vi "AlliGator Highlight Image ROI in Phasor Plot.vi"(0 "Source Image in":T1, 1 "Image Sum":T1, 2 "Source Image ROI Mask":T1, 5 "Phasor Plot Image in":T1, 7 "ROI":T2, 9 "[Corrected] Complex Phasor Array":csg[][](array[numeric]), 11 "Error In":errorcluster, 12 "Overlay Color":u32(colorbox), 13 "Phasor Plot Display Range":cluster{"Min Value":dbl, "Max Value":dbl}={"Min Value"=0.0, "Max Value"=nan}) -> (4 "Source Image out":T1, 6 "Phasor Plot Image out":T1, 10 "CPU (s)":dbl, 15 "Error Out":errorcluster)   [LabVIEW 2021, in "AlliGator Phasor Plot.lvlib"]
doc: "Highlights the phasors in the Phasor Plot image that corrspond to pixels in the Source Image ROI."
uses:
  AlliGator Phasor Plot.lvlib
  <vilib>/vision/Image Controls.llb/IMAQ Image.ctl
  Palette/Image Palette Information.ctl
  Image/Image Display Palette Type.ctl
  Globals, Variables, Constants/AlliGator Variables List.ctl
  Settings/AlliGator Settings List.ctl
  Phasor Ratio/AlliGator Phasor Plot Reference Points.ctl
  40af3798-00bb-4b94-b92d-50ae21bc0bc0.vi
  Image/Global Rectangle Origin & Size.vi
  Variant/Variant to Data/Variant to Boolean.vi
  Variant/Variant to Data/Variant to I32.vi
  Image/Image Get Pixel Color.vi
  Image/Adjust Pixel Overlay Brightness.vi
  Globals, Variables, Constants/AlliGator Globals, Variables & Constants.lvlib
  Phasor Ratio/AlliGator Phasor Ratio.lvlib
  Image/Image.lvlib
  Source Image/AlliGator Source Image.lvlib
  <vilib>/vision/NI_Vision_Development_Module.lvlib
  Error/Error.lvlib
  Time/Time.lvlib
  ROIs/AlliGator ROIs.lvlib
  Settings/AlliGator Settings.lvlib
  Variant/Variant to Data/Variant to Data.lvlib
  Palette/Palette.lvlib
panel:
  # "see the AlliGator License on the block diagram (Ctrl+E or Window:Show Block Diagram)"
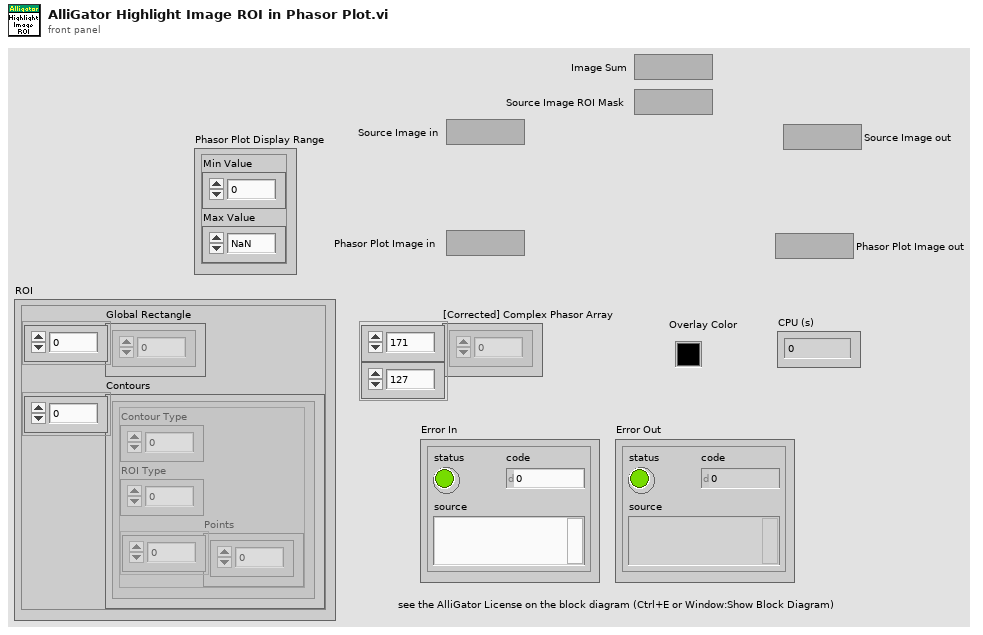
[diagram p1: front panel]
types:
  T1 = typedef "IMAQ Image.ctl" = refnum<image>
  T2 = cluster{"Global Rectangle":i32[], "Contours":cluster{"Contour Type":u32, "ROI Type":u32, "Points":i32[]}[]}
  T3 = typedef "Palette.lvlib/Image Palette Information.ctl" = cluster{"Palette Name [# Colors,int?,inv?]":string, "Palette Type":T4, "Palette Colors":u32[], "Interpolate?":bool}
  T4 = typedef "Image.lvlib/Image Display Palette Type.ctl" = u32
  T5 = typedef "AlliGator Globals, Variables & Constants.lvlib/AlliGator Variables List.ctl" = enum16{"---- GUI ----", "GUI:Initialization Status", "GUI:State Indicators Refnum", "GUI:Original AlliGator Menu Items", "GUI:Current Action Loop State", "GUI:Script in progress", "GUI:Playback", "GUI:Loop Playback", "GUI:Search ROI Used", "GUI:Search ROI", "Decay Graph Max Legend Size", "Intensity Graph Max Legend Size", "Decay Statistics Graph Max Legend Size", "Phasor Graph Max Legend Size", "Phasor Ratio Graph Max Legend Size", "Lifetime Graph Max Legend Size", "---- Files ----", "Files:Export Dataset Frames as Individual Files", "Files:Show Batch Export Help Balloons", "Files:Frames in Dataset", "Files:ptu File Frame Start Indices", "Files:Current Frame in Dataset", "Files:Current Frame Timestamp", "Files:Dataset Loaded", "Files:Dataset Metadata", "Files:Dataset Channel", "Files:Dataset Data Description", "Files:Background Dataset Metadata", "Files:Background Dataset Channel", "Files:Background Dataset Data Description", "Files:Background File Subtraction", "Files:Background File Path", "Files:Background File Pile-up Correction", "Files:Background File Pixel Well Capacity", "Files:Background File Scaling Factor", "Files:Current Dataset Load Settings", "Files:Dataset Path", "Files:ICCD-specific Information", "Files:Macrotime Gate Separation", "------ Python Plugins ------", "Python Plugins:Information", "Python Plugins:Python Session", "Python Plugins:Valid Python Session?", "---- Source Image ----", "Source Image:ROIs", "Source Image:Current ROI", "Source Image:ROI Event Refnum", "X_Source Image Display Range", "X_Source Image Palette Information", "X_Type of Displayed Image", "X_Time Gate Slider", "Source Image:Palette List", "Source Image:Scale", "Source Image:ROI Overlay Color", "Source Image:Overlay to Erase", "Source Image:Is Displayed Image Accumulated", "Source Image:White Light Image Modified", "Source Image:Mask Image Modified", "---- Image Profile Window ----", "Image Profile:Window Event Refnum", "Image Profile:IntensityType", "Image Profile:Intensity Average Type", "Image Profile:Intensity-weighted SDV", "Image Profile:Box Profile Type", "Image Profile:Window Open", "Image Profile:Plotted Fit Parameter", "------ Phasor Graph -------", "Phasor Graph:Show Line", "---- Phasor Plot ---", "Phasor Plot:Parameters Changed", "Phasor Plot:FLI Dataset Modified since last Calculation", "Phasor Harmonics Data", "Selected Phasor Harmonics", "Phasor Harmonic Manager Event Refnum", "Phasor Plot:ROIs", "Phasor Plot:Current ROI", "Phasor Plot:ROI Event Refnum", "Phasor Plot:Image Reference Points", "Phasor Plot:Computed", "Phasor Plot:Palette Information", "Phasor Plot:Palette List", "Phasor Plot:Phasor Ratio Palette Information", "Phasor Plot:Phasor Ratio Palette List", "Phasor Plot:Image Scale", "Phasor Plot:Image Overlay to Erase", "Phasor Plot:Image Elements to Update", "Phasor Plot:Current Calculation Parameters", "Phasor Plot:Current Calibration Options", "Phasor Plot:Reset Cumulated Phasor Plot", "Phasor Plot:Reference 1", "Phasor Plot:Lifetime Reference 1", "Phasor Plot:Reference 1 Frequency", "Phasor Plot:Reference 2", "Phasor Plot:Lifetime Reference 2", "Phasor Plot:Reference 2 Frequency", "---- Decay Analysis ----", "Number of Selected Decays to Fit", "LS Fit Results", "LAR Fit Results", "BS Fit Results", "Last Decay Max - Min", "Best Fit Parameters", "Best Fit Parameter Names", "Actual Size X", "Actual Size Y", "Binning X", "Binning Y", "Actual # Gates", "Dataset Number", "Gates to...", "Gates Skipped", "Gates to keep", "Gate Step", "Gate Separation", "Reversed Gates", "Pile-up Correction", "Pixel Well Capacity", "Background Subtracted", "Background Subtraction Method", "Background Definition Range", "Background File (deprecated)", "Number of Dataset Accumulated", "Array of Accumulated Dataset Paths", "Do Averaged Datasets", "Destination File Path", "Process Plot Target", "Use 1/D as Phasor Frequency", "---- Decay Fit Parameter Map -----", "Decay Fit Parameter Map:Palette Information", "Decay Fit Parameter Map:Palette List", "---- Parameter Map ----", "Parameter Map:Palette Information", "Parameter Map:Palette List", "------- Local Decay Window ---------", "Local Decay Graph Window:Event Refnum", "Local Decay Graph Window:Use normalized IRF for convolution", "----- Miscellaneous ----", "Misc:Skippable Dialog Windows Status"}
  T6 = typedef "AlliGator Settings.lvlib/AlliGator Settings List.ctl" = enum16{"GUI:Visible Settings Tab", "GUI:Last Run Version", "Source Image:Use Image Histogram for Contrast", "Source Image:Low Count Pixels Rejection Options", "Source Image:High Count Pixels Rejection Options", "Source Image:Use Image Brightness", "Source Image:Blend Overlay with Image Background", "Source Image:Use Fixed ROI Diameter", "Source Image:ROI Diameter", "Source Image:ROI Center Color", "Source Image:Peak Threshold", "Source Image:Intensity Threshold", "Source Image:Image Binning Options", "Source Image:Image Smoothing Options", "Source Image:Image Histogram Active", "Source Image:Invert Binary Mask", "Source Image:Hot Pixel Removal", "Source Image:Overlay Analyzed ROI Center", "Source Image:Auto-Adjust Contrast", "Source Image:Histogram Lower Percentile", "Source Image:Histogram Upper Percentile", "Source Image:Save Source Image", "Source Image:Scale Bar Options", "Source Image:Image Resolution (Pixel Size)", "Source Image:Flatfield Correction", "Source Image:Show Dead Left Columns Correction", "Source Image:Dead Left Columns Correction", "Source Image:Image Pre-Processing Operations Order", "Source Image:Overlay ROI Median", "Source Image:Median Overlay Color", "Data Information:Gate Width", "Data Information:Nanotime Gate Separation", "Data Information:Macrotime Gate Separation", "Data Information:Gate Step", "Data Information:# Gates", "Data Information:Gate Image Exposure", "Data Information:Gate Image Integration", "Data Information:Gates to Skip", "Data Information:Gates to Keep", "Data Information:Define Gates to", "Data Information:Channel Name", "Data Information:Available Channel Names", "Data Information:Channel Arithmetic", "Data Information:Background File Subtraction", "Data Information:Background File", "Data Information:Background Scaling Factor", "Data Information:Background Pile-up Correction", "Data Information:Background Pixel Well Capacity", "Data Information:Laser Period", "Data Information:SYNC Period", "Data Information:Pile-up Correction", "Data Information:Pixel Well Capacity", "Data Information:Dataset Scaling Factor", "Fluorescence Decay_Decay Pre-Processing:Reverse Gates", "Fluorescence Decay_Decay Pre-Processing:Verbose Decay Pre-Processing", "Fluorescence Decay_Decay Pre-Processing:Use Decay Pre-Processing", "Fluorescence Decay_Decay Pre-Processing:Background Subtraction", "Fluorescence Decay_Decay Pre-Processing:Background Definition Range", "Fluorescence Decay_Decay Pre-Processing:Baseline Subtraction Method", "Fluorescence Decay_Decay Pre-Processing:Decay Pre-Processing Operations Order", "Fluorescence Decay_Decay Pre-Processing:Smoothing Parameter", "Fluorescence Decay_Decay Pre-Processing:Shift Decay", "Fluorescence Decay_Decay Pre-Processing:Decay Shift Parameters", "Fluorescence Decay_Decay Pre-Processing:Fold Decay", "Fluorescence Decay_Decay Pre-Processing:# Folds", "Fluorescence Decay_Decay Pre-Processing:1-Normalize Decay", "Fluorescence Decay_Decay Pre-Processing:[0-1]-Normalize Decay", "Fluorescence Decay_Decay Pre-Processing:Smoothen Decay", "Fluorescence Decay_Decay Pre-Processing:Extrapolate Decay", "Fluorescence Decay_Decay Pre-Processing:Use Periodicity", "Fluorescence Decay_Decay Pre-Processing:Use Cursors", "Fluorescence Decay_Decay Pre-Processing:Tail Fraction", "Fluorescence Decay_Decay Pre-Processing:Head Fraction", "Fluorescence Decay_Decay Pre-Processing:Additional Points", "Fluorescence Decay_Decay Pre-Processing:Straighten Decay", "Fluorescence Decay_Decay Pre-Processing:Constant Background", "Fluorescence Decay_Decay Pre-Processing:Pixel-Normalize Decay", "Fluorescence Decay_Advanced Analysis:Extract IRF instead of Decay", "Fluorescence Decay_Advanced Analysis:IRF Extraction Options", "Fluorescence Decay_Advanced Analysis:IRF Optimization Options", "Fluorescence Decay_Advanced Analysis:Square Pulse Options", "Fluorescence Decay_Advanced Analysis:IRF Order", "Fluorescence Decay_Advanced Analysis:IRF Time Constants", "Fluorescence Decay_Advanced Analysis:Wavelet Analysis Options", "Fluorescence Decay_Advanced Analysis:Average Lifetime Options", "Fluorescence Decay_Fit Options:Fit Options", "Fluorescence Decay_Fit Options:Use Legacy Fitting Approach", "Fluorescence Decay_Fit Options:Use Data Information Laser Period", "Fluorescence Decay_Fit Parameters:Displayed Fit Parameters", "Fluorescence Decay_Fit Parameters:Fit Parameter Constraints", "Fluorescence Decay_Fit Parameters:Export Tabulated Results", "Fluorescence Decay_Fit Parameters:MLE Baseline Offset Type", "Fluorescence Decay_Fit Parameters:MLE Baseline Offset", "Fluorescence Decay_Fit Parameters:Guess Parameter Names", "Fluorescence Decay_Fit Parameters:Guess Parameter Values", "Fluorescence Decay_Fit Parameters:Guess Parameters Options", "Fluorescence Decay_Styles:Show Last Decay Only", "Fluorescence Decay_Styles:Decay Graph Color Array", "Fluorescence Decay:Decay Graph Active", "Fluorescence Decay Statistics:Min Peak Value", "Fluorescence Decay Statistics:Reject Low Decay Peak Pixels", "Fluorescence Decay Statistics:Reject High Decay Peak Pixels", "Fluorescence Decay Statistics:Max Peak Value", "Time Traces:Use File Timestamp", "Time Traces:Time Step", "Time Traces:Use Intensity Correction File", "Time Traces:Intensity Correction File", "Phasor Plot:Phasor Plot Smoothing Options", "Phasor Plot:Phasor Plot Size", "Phasor Plot:Phasor Plot Graphics Options", "Phasor Plot:Cumulative Phasor Plot", "Phasor Plot:Use Phasor Brightness", "Phasor Plot:Blend Overlay with Phasor Background", "Phasor Plot:Save Phasor Plot", "Phasor Plot:Show References", "Phasor Plot:Phasor Ratio Decay Range", "Phasor Plot:Exponential Fading", "Phasor Plot:Phasor Ratio Reference Colors", "Phasor Plot:Reference Radius", "Phasor Plot:Show Color Map Vertices", "Phasor Plot:Phasor Plot Active", "Phasor Plot:Phasor Ratio Color Map Type", "Phasor Plot:Phasor Ratio Color Map", "Phasor Plot:Phasor Ratio Display Range", "Phasor Plot:Selected Image ROI(s)", "Phasor Plot:All Image ROIs", "Phasor Plot:Selected Phasor Plot ROI(s)", "Phasor Plot:All Phasor Plot ROIs", "Phasor Plot:Phasor Ratio Color-Coded Quantity", "Phasor Plot:Store Phasor Harmonics", "Phasor Plot:Draw Reference Segment", "Phasor Plot:User-Defined Quantity", "Phasor Graph:Phasor Frequency", "Phasor Graph:Phasor Ratio Type", "Phasor Graph:Pixel-level Phasor Computation", "Phasor Graph:Save Phasor Graph", "Phasor Graph:Phasor Graph Active", "Phasor Graph:Phasor SDV Options", "Phasor Calibration:Use Backup Calibration if needed", "Phasor Graph:Define Shortest Lifetime as", "Phasor Calibration:Backup Calibration Type", "Phasor Calibration:Calibration Type", "Phasor Calibration:Calibration Lifetime", "Phasor Calibration:Calibration Map Algorithm", "Single-Exponential Phasor Locus (SEPL):Gate Parameters", "Single-Exponential Phasor Locus (SEPL):User-defined Gate", "Single-Exponential Phasor Locus (SEPL):User-defined IRF", "Single-Exponential Phasor Locus (SEPL):Phasor Parameters", "Single-Exponential Phasor Locus (SEPL):Decay & IRF Parameters", "Single-Exponential Phasor Locus (SEPL):Display Parameters", "Lifetime Analysis:Decay Analysis Parameters", "Lifetime Analysis:Lifetime Map Active", "Plugins:Python Settings", "Miscellaneous:Verbose Mode", "Miscellaneous:Beep after Script", "Miscellaneous:Saved Image File Format", "Miscellaneous:Exported Gate Image Settings", "Miscellaneous:Include Loading in Timing", "Miscellaneous:Verbose Settings Mode", "Miscellaneous:Histogram Options", "Miscellaneous:Beep on Error", "Miscellaneous:# Logical Processors Used", "Miscellaneous:ROI Description Max Characters", "Miscellaneous:Verbose Error Mode", "Miscellaneous:Transparent Mask Color"}
  T7 = typedef "AlliGator Phasor Ratio.lvlib/AlliGator Phasor Plot Reference Points.ctl" = cluster{"O_h":dbl, "O_v":dbl, "1_h":dbl, "1_v":dbl}
  T8 = typedef "ROI Descriptor" = cluster{"Global Rectangle":i32[], "Contours":cluster{"ID":enum32{"External", "Internal"}, "Type":u32, "Coordinates":i32[]}[]}
  T9 = cluster{"Red (or Hue) value":u8, "Green (or Sat) value":u8, "Blue (or Light or Val) value":u8}
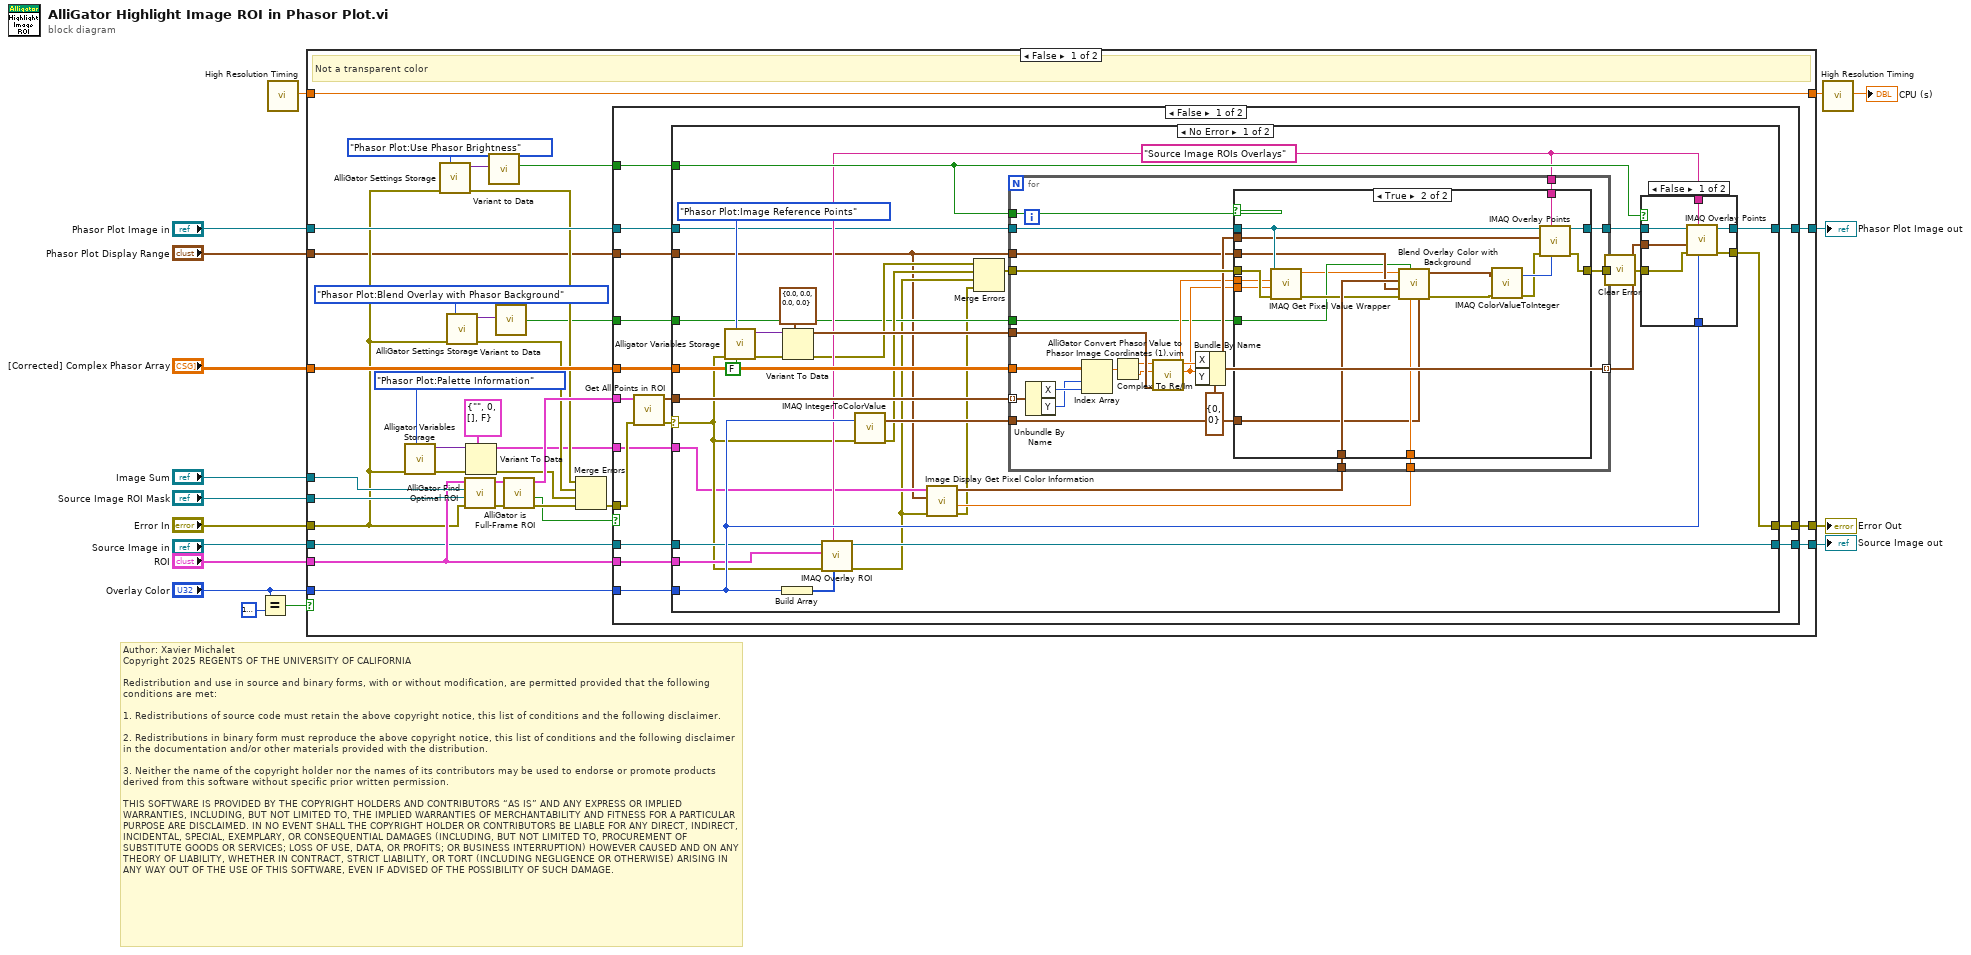
[diagram p0: block diagram]
diagram:
  # "Author: Xavier Michalet\nCopyright 2025 REGENTS OF THE UNIVERSITY OF CALIFORNIA\n\nRedistribution and use in source and binary forms, with or without modification, are permitted provided that the following conditions are met:\n\n1. Redistributions of source code must retain the above copyright notice, this list of conditions and the following disclaimer.\n\n2. Redistributions in binary form must reproduce the above copyright notice, this list of conditions and the following disclaimer in the documentation and/or other materials provided with the distribution.\n\n3. Neither the name of the copyright holder nor the names of its contributors may be used to endorse or promote products derived from this software without specific prior written permission.\n\nTHIS SOFTWARE IS PROVIDED BY THE COPYRIGHT HOLDERS AND CONTRIBUTORS “AS IS” AND ANY EXPRESS OR IMPLIED WARRANTIES, INCLUDING, BUT NOT LIMITED TO, THE IMPLIED WARRANTIES OF MERCHANTABILITY AND FITNESS FOR A PARTICULAR PURPOSE ARE DISCLAIMED. IN NO EVENT SHALL THE COPYRIGHT HOLDER OR CONTRIBUTORS BE LIABLE FOR ANY DIRECT, INDIRECT, INCIDENTAL, SPECIAL, EXEMPLARY, OR CONSEQUENTIAL DAMAGES (INCLUDING, BUT NOT LIMITED TO, PROCUREMENT OF SUBSTITUTE GOODS OR SERVICES; LOSS OF USE, DATA, OR PROFITS; OR BUSINESS INTERRUPTION) HOWEVER CAUSED AND ON ANY THEORY OF LIABILITY, WHETHER IN CONTRACT, STRICT LIABILITY, OR TORT (INCLUDING NEGLIGENCE OR OTHERWISE) ARISING IN ANY WAY OUT OF THE USE OF THIS SOFTWARE, EVEN IF ADVISED OF THE POSSIBILITY OF SUCH DAMAGE."
  n1 = Equal?(x="Overlay Color", y=u32 16777216 ("Overlay Color")) -> (x = y?=w10:bool)
  n2 = call "High Resolution Timing.vi"() -> ("elapsed (relative) seconds"=w12:dbl)  [unwired: 17 in, 2 out]
  n3 = case shown="False" w10 {
    tunnel: "[Corrected] Complex Phasor Array" -> [w50 _]
    tunnel: "Error In" -> [w22 w162]
    tunnel: [w38 w162] -> w15
    tunnel: "Image Sum" -> [w49 _]
    tunnel: "Overlay Color" -> [w48 _]
    tunnel: w12 -> [w47 w161]
    tunnel: [w47 w161] -> w11
    tunnel: "Source Image ROI Mask" -> [w46 _]
    tunnel: "Phasor Plot Image in" -> [w43 w160]
    tunnel: [w42 w160] -> w6
    tunnel: "ROI" -> [w41 _]
    tunnel: "Source Image in" -> [w40 w159]
    tunnel: [w39 w159] -> w3
    tunnel: "Phasor Plot Display Range" -> [w18 _]
    frame False {
      # "Not a transparent color"
      n4 = call "Alligator Variables Storage.vi"("AlliGator Variable"=AlliGator_Variables_List."Phasor Plot:Palette Information" ("Alligator Variable"), "Error In"=w22) -> ("Error Out"=w21:errorcluster, "Data out"=w25:variant)  [unwired: 7 in, 1 out]
      n5 = call "AlliGator Settings Storage.vi"("AlliGator Settings List"=AlliGator_Settings_List."Phasor Plot:Use Phasor Brightness", "Error In"=w22) -> ("Error Out"=w31:errorcluster, "Variant Data out"=w34:variant)  [unwired: 8 in]
      n6 = call "AlliGator Settings Storage.vi"("AlliGator Settings List"=AlliGator_Settings_List."Phasor Plot:Blend Overlay with Phasor Background", "Error In"=w22) -> ("Error Out"=w27:errorcluster, "Variant Data out"=w28:variant)  [unwired: 8 in]
      n7 = call "AlliGator Find Optimal ROI.vi"("error in (no error)"=w22, "ROI Mask"=w46, "Image Sum"=w49, "ROI Descriptor in"=w41) -> ("error out"=w45:errorcluster, "ROI Descriptor out"=w44:T8)  [unwired: 5 in, 1 out]
      n8 = Variant To Data(error in=w21, type=T3 {"Palette Name [# Colors,int?,inv?]"="", "Palette Type"=0, "Palette Colors"=[], "Interpolate?"=FALSE} ("Image Display Palette Information"), Variant=w25) -> (data=w19:T3, error out=w20:errorcluster)
      n9 = call-poly "Variant to Data.vi"("Variant"=w34) -> ("Value"=w33:bool)  [unwired: 8 in]
      n10 = call-poly "Variant to Data.vi"("Variant"=w28) -> ("Value"=w26:bool)  [unwired: 8 in]
      n11 = call "AlliGator is Full-Frame ROI.vi"("error in (no error)"=w45, "ROI Descriptor in"=w44) -> ("error out"=w37:errorcluster, "Full-Frame ROI?"=w35:bool, "ROI Descriptor (dup)"=w36:T8)  [unwired: 7 in]
      n12 = Merge Errors(w31, w27, w20, w37) -> (w32:errorcluster)
      n13 = case shown="False" w35 {
        tunnel: w50 -> [w66 _]
        tunnel: w33 -> [w65 _]
        tunnel: w48 -> [w64 _]
        tunnel: w43 -> [w61 w156]
        tunnel: [w60 w156] -> w42
        tunnel: w41 -> [w59 _]
        tunnel: w40 -> [w58 w157]
        tunnel: [w57 w157] -> w39
        tunnel: [w56 w158] -> w38
        tunnel: w32 -> [w55 w158]
        tunnel: w36 -> [w54 _]
        tunnel: w26 -> [w53 _]
        tunnel: w19 -> [w52 _]
        tunnel: w18 -> [w51 _]
        frame False {
          n14 = call "Get All Points in ROI.vi"("Error In"=w55, "ROI Descriptor"=w54) -> ("Error Out"=w62:errorcluster, "Point Array"=w63:cluster{"X":i32, "Y":i32}[])  [unwired: 8 in]
          n15 = case shown="No Error" w62 {
            selector: w62 -> [w74 _]
            tunnel: w66 -> [w100 _]
            tunnel: w65 -> [w99 _]
            tunnel: w64 -> [w98 _]
            tunnel: w59 -> [w97 _]
            tunnel: w63 -> [w89 _]
            tunnel: w61 -> [w79 w154]
            tunnel: [w78 w154] -> w60
            tunnel: w58 -> [w77 w155]
            tunnel: [w76 w155] -> w57
            tunnel: [w75 _] -> w56
            tunnel: w53 -> [w73 _]
            tunnel: w52 -> [w72 _]
            tunnel: w51 -> [w67 _]
            frame No Error {
              w84 = "Source Image ROIs Overlays" ("Group")
              n16 = call "Alligator Variables Storage.vi"("Get(F)/Set"=FALSE, "AlliGator Variable"=AlliGator_Variables_List."Phasor Plot:Image Reference Points" ("Alligator Variable"), "Error In"=w74) -> ("Error Out"=w92:errorcluster, "Data out"=w94:variant)  [unwired: 6 in, 1 out]
              n17 = Build Array(w98) -> (w90:u32[])
              n18 = Variant To Data(error in=w92, type=T7 {"O_h"=0.0, "O_v"=0.0, "1_h"=0.0, "1_v"=0.0} ("Phasor Plot Reference Points"), Variant=w94) -> (data=w91:T7, error out=w81:errorcluster)
              n19 = call "IMAQ Overlay ROI"("Colors (Green)"=w90, "Group"=w84, "error in (no error)"=w74, "ROI Descriptor"=w97, "Image"=w77) -> ("error out"=w69:errorcluster, "Image Out"=w76:T1)  [unwired: 5 in]
              n20 = call "IMAQ IntegerToColorValue"("error in (no error)"=w74, "U32 value"=w98) -> ("error out"=w80:errorcluster, "Color Value"=w85:T9)  [unwired: 3 in, 2 out]
              n21 = call "Image Display Get Pixel Color Information.vi"("Error In"=w69, "Image Display Range"=w67, "Image Display Palette Information"=w72) -> ("Error Out"=w68:errorcluster, "Image Scale Factor (256 colors)"=w70:sgl, "1D Color Array"=w71:cluster{"Red":u8, "Green":u8, "Blue":u8}[])  [unwired: 5 in, 1 out]
              n22 = Merge Errors(w81, w80, w69, w68) -> (w82:errorcluster)
              n23 = for {
                tunnel: w100 -> [w132]
                tunnel: w91 -> [w131]
                tunnel: w89 -> [w129] mode=indexing
                tunnel: [w120] -> w88 mode=indexing
                tunnel: w99 -> [w125]
                tunnel: w85 -> [w114]
                tunnel: w84 -> [w119]
                tunnel: w82 -> [w122]
                tunnel: [w121] -> w86
                tunnel: w79 -> [w124]
                tunnel: [w123] -> w87
                tunnel: w73 -> [w113]
                tunnel: w71 -> [w112]
                tunnel: w70 -> [w111]
                tunnel: w67 -> [w110]
                n24 = Unbundle By Name(w129) -> ("X"=w116:i32, "Y"=w115:i32)
                n25 = Index Array(array=w132, index (row)=w115, index (col)=w116) -> (element=w130:csg)
                n26 = Complex To Re/Im(x + iy=w130) -> (x=w128:sgl, y=w127:sgl)
                n27 = call "AlliGator Convert Phasor Value to Phasor Image Coordinates (1).vim"("Phasor Plot Reference Points"=w131, "Phasor s"=w127, "Phasor g"=w128) -> ("Phasor Plot y"=w117:dbl, "Phasor Plot x"=w118:dbl)  [unwired: 7 in]
                n28 = Bundle By Name(cluster=cluster{"X":i32, "Y":i32} {"X"=0, "Y"=0} ("Point"), "X"=w118, "Y"=w117) -> (w120:cluster{"X":i32, "Y":i32})
                n29 = case shown="True" w125 {
                  tunnel: w124 -> [w134 w151]
                  tunnel: [w134 w153] -> w123
                  tunnel: w122 -> [w133 w152]
                  tunnel: [w133 w147] -> w121
                  tunnel: w120 -> [_ w150]
                  tunnel: w119 -> [_ w146]
                  tunnel: w118 -> [_ w145]
                  tunnel: w117 -> [_ w144]
                  tunnel: w114 -> [_ w137]
                  tunnel: w113 -> [_ w139]
                  tunnel: w112 -> [_ w143]
                  tunnel: w111 -> [_ w138]
                  tunnel: w110 -> [_ w142]
                  frame False {
                  }
                  frame True {
                    n30 = call "IMAQ Get Pixel Value Wrapper.vi"("Error In"=w152, "Y Coordinate"=w144, "X Coordinate"=w145, "Image"=w151) -> ("Error Out"=w141:errorcluster, "Pixel Value"=w136:sgl)  [unwired: 5 in, 1 out]
                    n31 = call "Blend Overlay Color with Background.vi"("Overlay Color Value"=w137, "Image Scale Factor"=w138, "Blend Overlay with Background"=w139, "error in (no error)"=w141, "Image Display Range"=w142, "Image Color Array"=w143, "Pixel Value"=w136) -> ("error out"=w140:errorcluster, "Scaled/Blended Overlay Color Value"=w135:T9)  [unwired: 3 in]
                    n32 = call "IMAQ ColorValueToInteger"("error in (no error)"=w140, "Color Value"=w135) -> ("error out"=w148:errorcluster, "U32 value"=w149:u32)  [unwired: 3 in, 2 out]
                    n33 = call "IMAQ Overlay Points"("Color"=w149, "Group"=w146, "error in (no error)"=w148, "Point"=w150, "Image"=w151) -> ("error out"=w147:errorcluster, "Image Out"=w153:T1)  [unwired: 5 in]
                  }
                }
              }
              n34 = call "Clear Error.vi"("Error In"=w86) -> ("no Error Out"=w83:errorcluster)  [unwired: 8 in]
              n35 = case shown="False" w99 {
                tunnel: w87 -> [w107 w109]
                tunnel: [w106 w109] -> w78
                tunnel: [w105 w108] -> w75
                tunnel: w84 -> [w104 _]
                tunnel: w98 -> [w103 _]
                tunnel: w88 -> [w102 _]
                tunnel: w83 -> [w101 w108]
                frame False {
                  n36 = call "IMAQ Overlay Points"("Color"=w103, "Group"=w104, "error in (no error)"=w101, "Array of Points"=w102, "Image"=w107) -> ("error out"=w105:errorcluster, "Image Out"=w106:T1)  [unwired: 5 in]
                }
                frame True {
                  # "this has been computed in the main For Loop"
                }
              }
            }
            frame Error {
              # "empty or no ROI"
            }
          }
        }
        frame True {
        }
      }
    }
    frame True {
    }
  }
  "Error Out" <- w15
  "Phasor Plot Image out" <- w6
  "Source Image out" <- w3
  n37 = call "High Resolution Timing.vi"("relative seconds (NaN)"=w11) -> ("elapsed (relative) seconds"=→"CPU (s)":dbl)  [unwired: 16 in, 2 out]
